vi "Get Object (RAW data).vi"(4 "Region":T1, 6 "Version ID":string, 7 "Request Parameters":T2, 8 "error in (no error)":errorcluster, 9 "Bucket":string, 10 "Object Path":string) -> (0 "error out":errorcluster, 2 "GetObjectResult":T4, 3 "Data":string)   [LabVIEW 2015, in "LV Interface for Amazon S3.lvlib"]
doc: "This operation <B>retrieves an object</B> from Amazon S3 <B> and returns RAW data. You must have READ access</B> to the object. If you grant READ access to the anonymous user, you can return the object without using an authorization header. To distribute large files to many people, you can <B>save bandwidth costs using BitTorrent</B>. You can <B>limit returned data using Request parameters</B>."
uses:
  LV Interface for Amazon S3.lvlib
  Typedefs/AMZ_S3_API_GETObjectResult.ctl
  Typedefs/AMZ_S3_API_GET Object Request Parameters.ctl
  Typedefs/AMZ_S3_API_GET Request Range.ctl
  Typedefs/AMZ_S3_LocationConstraint.ctl
  Typedefs/AMZ_S3_Call Results.ctl
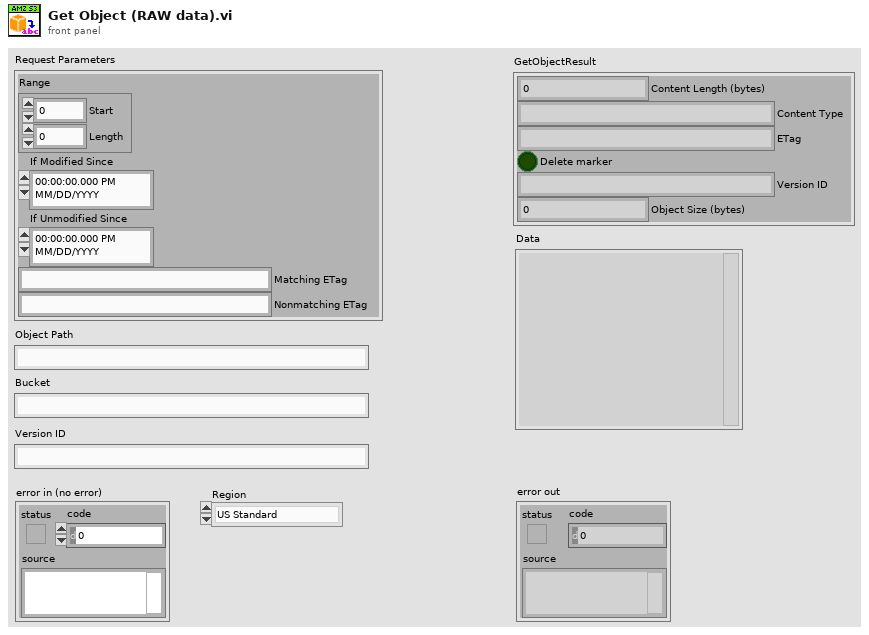
[diagram p1: front panel]
types:
  T1 = typedef "LV Interface for Amazon S3.lvlib/AMZ_S3_LocationConstraint.ctl" = enum16{"US Standard", "us-east-2", "us-west-1", "us-west-2", "ap-northeast-1", "ap-northeast-2", "ap-southeast-1", "ap-southeast-2", "ca-central-1", "eu-central-1", "eu-west-1", "eu-west-2", "sa-east-1"}
  T2 = typedef "LV Interface for Amazon S3.lvlib/AMZ_S3_API_GET Object Request Parameters.ctl" = cluster{"Range":T3, "If Modified Since":timestamp, "If Unmodified Since":timestamp, "Matching ETag":string, "Nonmatching ETag":string}
  T3 = typedef "LV Interface for Amazon S3.lvlib/AMZ_S3_API_GET Request Range.ctl" = cluster{"Start":i64, "Length":i64}
  T4 = typedef "LV Interface for Amazon S3.lvlib/AMZ_S3_API_GETObjectResult.ctl" = cluster{"Content Length (bytes)":u64, "Content Type":string, "ETag":string, "Delete marker":bool, "Version ID":string, "Object Size (bytes)":u64}
  T5 = typedef "LV Interface for Amazon S3.lvlib/AMZ_S3_Call Results.ctl" = enum16{"Success", "UndefinedError", "AccessDenied", "AccountProblem", "AmbiguousGrantByEmailAddress", "BadDigest", "BucketAlreadyExists", "BucketAlreadyOwnedByYou", "BucketNotEmpty", "CredentialsNotSupported", "CrossLocationLoggingProhibited", "EntityTooSmall", "EntityTooLarge", "ExpiredToken", "IllegalVersioningConfigurationException", "IncompleteBody", "IncorrectNumberOfFilesInPostRequest", "InlineDataTooLarge", "InternalError", "InvalidAccessKeyId", "InvalidAddressingHeader", "InvalidArgument", "InvalidBucketName", "InvalidDigest", "InvalidLocationConstraint", "InvalidPart", "InvalidPartOrder", "InvalidPayer", "InvalidPolicyDocument", "InvalidRange", "InvalidSecurity", "InvalidSOAPRequest", "InvalidStorageClass", "InvalidTargetBucketForLogging", "InvalidToken", "InvalidURI", "KeyTooLong", "MalformedACLError", "MalformedPOSTRequest", "MalformedXML", "MaxMessageLengthExceeded", "MaxPostPreDataLengthExceededError", "MetadataTooLarge", "MethodNotAllowed", "MissingAttachment", "MissingContentLength", "MissingRequestBodyError", "MissingSecurityElement", "MissingSecurityHeader", "NoLoggingStatusForKey", "NoSuchBucket", "NoSuchKey", "NoSuchUpload", "NoSuchVersion", "NotImplemented", "NotSignedUp", "OperationAborted", "PermanentRedirect", "PreconditionFailed", "Redirect", "RequestIsNotMultiPartContent", "RequestTimeout", "RequestTimeTooSkewed", "RequestTorrentOfBucketError", "SignatureDoesNotMatch", "SlowDown", "TemporaryRedirect", "TokenRefreshRequired", "TooManyBuckets", "UnexpectedContent", "UnresolvableGrantByEmailAddress", "UserKeyMustBeSpecified", "LabVIEWError"}
  T6 = typedef "LV Interface for Amazon S3.lvlib/AMZ_S3_HTTP Header-Value pair.ctl" = cluster{"Header":string, "Value":string}
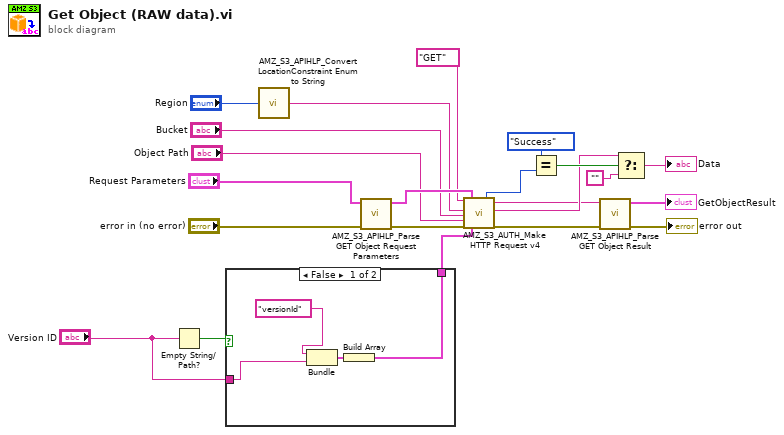
[diagram p0: block diagram]
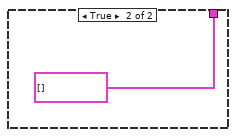
[diagram p2: hidden frame]
diagram:
  n1 = Empty String/Path?(string/path="Version ID") -> (empty?=w12:bool)
  n2 = case shown="False" w12 {
    tunnel: [w23 cluster{"item":string, "value":string}[] [] ("request parameters")] -> w7
    tunnel: "Version ID" -> [w26 _]
    frame False {
      n3 = Bundle("versionId", "Version ID"=w26) -> (w24:cluster{string, "Version ID":string})  [unwired: 1 in]
      n4 = Build Array(w24) -> (w23:cluster{string, "Version ID":string}[])
    }
    frame True {
    }
  }
  n5 = call "AMZ_S3_APIHLP_Convert LocationConstraint Enum to String.vi"("Location"="Region") -> ("Location String"=w1:string)  [unwired: 4 in]
  n6 = call "AMZ_S3_APIHLP_Parse GET Object Request Parameters.vi"("GET Object Request Parameters"="Request Parameters", "error in (no error)"="error in (no error)") -> ("error out"=w22:errorcluster, "HTTP Headers"=w8:T6[])  [unwired: 8 in]
  n7 = call "AMZ_S3_AUTH_Make HTTP Request v4.vi"("HTTP-Verb"="GET", "Region"=w1, "Bucket"="Bucket", "Object Key"="Object Path", "error in"=w22, "request headers"=w8, "request parameters"=w7) -> ("Call Result"=w9:T5, "response headers"=w10:string, "response body"=w17:string, "error out"=w15:errorcluster)  [unwired: 9 in]
  n8 = Equal?(x=AMZ_S3_Call_Results."Success" ("y"), y=w9) -> (x = y?=w18:bool)
  n9 = call "AMZ_S3_APIHLP_Parse GET Object Result.vi"("error in (no error)"=w15, "Response header"=w10) -> ("error out"=→"error out":errorcluster, "GetObjectResult"=→"GetObjectResult":T4)  [unwired: 8 in]
  n10 = Select(t=w17, s=w18, f="") -> (s? t:f=→"Data":string)
